vi "class_data.vi"() -> ()   [LabVIEW 2010, in "DataCollectionDL091104Scaffold.lvclass"]
uses:
  DataCollectionDL091104Scaffold.lvclass
panel:
  in  "file name base":string
  in  "data folder path":path
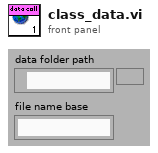
[diagram p1: front panel]
diagram:
